vi "LV SciSDK OSCILLOSCOPE ARM.vi"(8 "error in (no error)":errorcluster, 9 "Oscilloscope Handle In":T2) -> (0 "error out":errorcluster, 1 "Oscilloscope Handle Out":T2)   [LabVIEW 2021, in "SciSDK_Labview.lvlib"]
uses:
  SciSDK_Labview.lvlib
panel:
  out "NI Error Code":i32
  in  "Board Handle In":T1
  out "Board Handle Out":T1
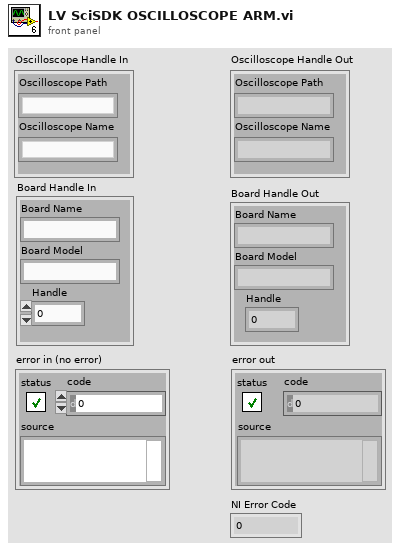
[diagram p1: front panel]
types:
  T1 = cluster{"Board Name":string, "Board Model":string, "Handle":u64}
  T2 = cluster{"Oscilloscope Path":string, "Oscilloscope Name":string}
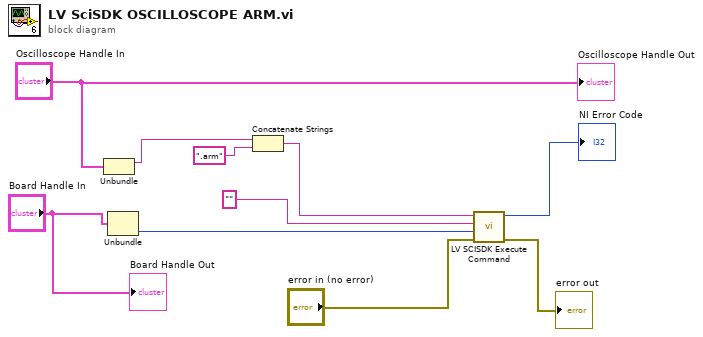
[diagram p0: block diagram]
diagram:
  n1 = Unbundle("Oscilloscope Handle In") -> ("Oscilloscope Path"=w3:string)  [unwired: 1 out]
  n2 = Unbundle("Board Handle In") -> ("Handle"=w1:u64)  [unwired: 2 out]
  n3 = Concatenate Strings(w3, ".arm" ("string")) -> (w8:string)
  n4 = call "LV SCISDK Execute Command.vi"("error in (no error)"="error in (no error)", "handle"=w1, "value"="", "Path"=w8) -> ("error out"=→"error out":errorcluster, "function return"=→"NI Error Code":i32)  [unwired: 5 in, 1 out]
  "Oscilloscope Handle Out" <- "Oscilloscope Handle In"
  "Board Handle Out" <- "Board Handle In"
